vi "Basic trigo.vi"() -> ()   [LabVIEW 2012]
uses:
  Motors Values.vi
panel:
  in  "Distance from camera":dbl
  out "Delta hieght":dbl
  in  "Camera offset Y":dbl
  out "Distance on ground":dbl
  in  "Caamera offset X":dbl
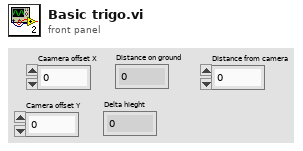
[diagram p1: front panel]
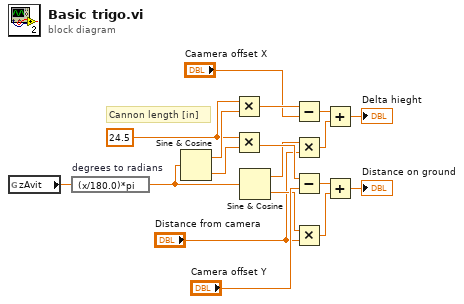
[diagram p0: block diagram]
diagram:
  w17 = 24.5
  # "Cannon length [in]"
  n1 = global read "Motors Values.vi" "zAvit"() -> (w15:dbl)
  n2 = expression code="(x/180.0)*pi" "degrees to radians"(w15) -> (w14:dbl)
  n3 = Sine & Cosine(0:w14) -> (1:w18:dbl, 2:w16:dbl)
  n4 = Multiply(x=w17, y=w18) -> (x*y=w13:dbl)
  n5 = Multiply(x=w17, y=w16) -> (x*y=w10:dbl)
  n6 = Sine & Cosine(0:w14) -> (1:w9:dbl, 2:w8:dbl)
  n7 = Subtract(x=w13, y="Caamera offset X") -> (x-y=w6:dbl)
  n8 = Multiply(x=w9, y="Distance from camera") -> (x*y=w5:dbl)
  n9 = Subtract(x=w10, y="Camera offset Y") -> (x-y=w2:dbl)
  n10 = Multiply(x=w8, y="Distance from camera") -> (x*y=w1:dbl)
  n11 = Add(x=w6, y=w5) -> (x+y=→"Delta hieght":dbl)
  n12 = Add(x=w2, y=w1) -> (x+y=→"Distance on ground":dbl)
